vi "GenerateWellCoordinates.vi"(10 "Columns":i32, 11 "Rows":i32) -> (3 "Well Coordinates":string)   [LabVIEW 2014]
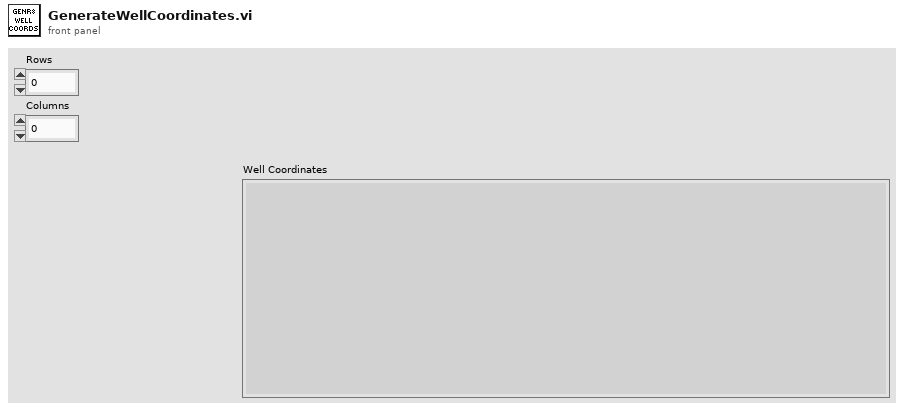
[diagram p1: front panel]
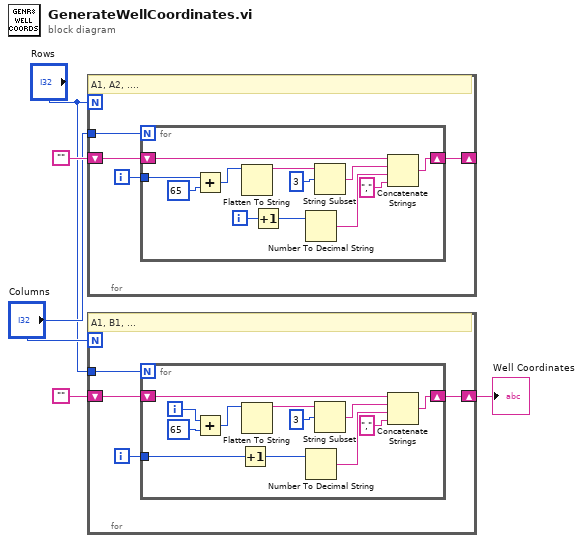
[diagram p0: block diagram]
diagram:
  n1 = for {
    N: "Rows" -> [_]
    tunnel: "Columns" -> [w9]
    shift-right: [w6] -> _
    shift-left: "" -> [w7]
    i -> [w8]
    # "A1, A2, ...."
    n2 = for {
      N: w9 -> [_]
      tunnel: w8 -> [w20]
      shift-right: [w13] -> w6
      shift-left: w7 -> [w14]
      i -> [w21]
      n3 = Add(x=w20, y=65) -> (x+y=w18:i32)
      n4 = Flatten To String(anything=w18) -> (data string=w12:string)  [unwired: 3 in, 2 out]
      n5 = Increment(x=w21) -> (x+1=w17:i32)
      n6 = Number To Decimal String(number=w17) -> (decimal integer string=w16:string)  [unwired: 1 in]
      n7 = String Subset(string=w12, offset (0)=3) -> (substring=w11:string)  [unwired: 1 in]
      n8 = Concatenate Strings(w14, w11, w16, "," ("string")) -> (w13:string)
    }
  }
  n9 = for {
    N: "Columns" -> [_]
    tunnel: "Rows" -> [w25]
    shift-right: [w22] -> w4
    shift-left: "" -> [w23]
    i -> [w24]
    # "A1, B1, ..."
    n10 = for {
      N: w25 -> [_]
      tunnel: w24 -> [w26]
      shift-right: [w31] -> w22
      shift-left: w23 -> [w32]
      i -> [w27]
      n11 = Add(x=w27, y=65) -> (x+y=w36:i32)
      n12 = Increment(x=w26) -> (x+1=w35:i32)
      n13 = Flatten To String(anything=w36) -> (data string=w30:string)  [unwired: 3 in, 2 out]
      n14 = Number To Decimal String(number=w35) -> (decimal integer string=w34:string)  [unwired: 1 in]
      n15 = String Subset(string=w30, offset (0)=3) -> (substring=w29:string)  [unwired: 1 in]
      n16 = Concatenate Strings(w32, w29, w34, "," ("string")) -> (w31:string)
    }
  }
  "Well Coordinates" <- w4
